vi "Close.vi"(8 "error in (no error)":errorcluster, 11 "Fetch Waveform CFG in":refnum<class "Fetch Waveforms CFG.lvclass">) -> (0 "error out":errorcluster, 3 "Fetch Waveform CFG out":refnum<class "Fetch Waveforms CFG.lvclass">)   [LabVIEW 2023, in "PXIe-4353.lvlib" / "Fetch Waveforms CFG.lvclass"]
uses:
  Fetch Waveforms CFG.lvclass
  Thermometer/Thermometer DAQmx/Thermometer DAQmx Config/Thermometer DAQmx Config.lvclass/Thermometer DAQmx Config.ctl
  Fetch Waveforms CFG.lvclass/Fetch Waveforms CFG.ctl
  Thermometer/Thermometer DAQmx/Thermometer DAQmx Config/Thermometer DAQmx Config.lvclass
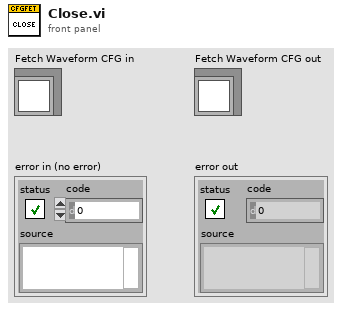
[diagram p1: front panel]
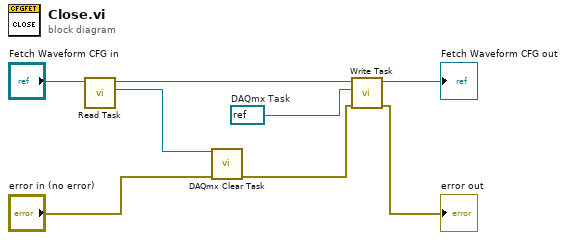
[diagram p0: block diagram]
diagram:
  w3 = refnum<k21> refnum  # DAQmx Task
  n1 = call "Read Task.vi"("Thermometer DAQmx Config in"="Fetch Waveform CFG in") -> ("Task"=w6:refnum<k21>, "Thermometer DAQmx Config out"=w7:refnum<class "Fetch Waveforms CFG.lvclass">)  [unwired: 8 in, 1 out]
  n2 = call <vilib>:"DAQmx Clear Task.vi"("task in"=w6, "error in"="error in (no error)") -> ("error out"=w2:errorcluster)  [unwired: 13 in]
  n3 = call "Write Task.vi"("error in (no error)"=w2, "Task"=w3, "Thermometer DAQmx Config in"=w7) -> ("error out"=→"error out":errorcluster, "Thermometer DAQmx Config out"=→"Fetch Waveform CFG out":refnum<class "Fetch Waveforms CFG.lvclass">)  [unwired: 7 in]
